vi "Controlador_PID.vi"() -> ()   [LabVIEW 2016]
uses:
  <vilib>/imath/engines/lvmath2/RunTimeEngine/Managers/WorkSpace/UID Generator.vi
  <vilib>/imath/engines/lvmath2/RunTimeEngine/RunTimeType/NIMS_RunTimeType_From StrictType (excl LVString).vi
  <instcachedir>/0/NIMS_RunTimeType_From StrictType (excl LVString)_BBF44FB49F834B71AF7A14CCEDF8BECD.lvgen/NIMS_RunTimeType_From StrictType (excl LVString)_BBF44FB49F834B71AF7A14CCEDF8BECD_000.vi
  <vilib>/imath/engines/lvmath2/RunTimeEngine/LocalVariableDefStatement/MC_LocalVariableDefStatement_Display.vi
  <vilib>/imath/engines/lvmath2/RunTimeEngine/Managers/SymbolTable/Clear UID.vi
  <vilib>/imath/engines/lvmath2/RunTimeEngine/NodeEndStatement/NIMS_NodeEndStatement_Output.vi
  <instcachedir>/0/NIMS_NodeEndStatement_Output_53EC0D466D134D7ABD903AC30B43404B.lvgen/NIMS_NodeEndStatement_Output_53EC0D466D134D7ABD903AC30B43404B_001.vi
  <vilib>/imath/engines/lvmath2/RunTimeEngine/ErrorHandling/NIMS_Finalize Error.vi
  <vilib>/imath/engines/lvmath2/RunTimeEngine/Managers/SymbolTable/NIMS_WorkSpace.lvlib
panel:
  in  "Ki":dbl=1.0
  in  "Kd":dbl=1.0
  in  "Kp":dbl=1.0
  in  "SP":dbl(knob)=1.0 scale=0.0..10.0
  in  "stop":bool
  out "Waveform Chart":cluster{"SP":dbl, "x":dbl}(graph)
  in  "F":dbl=1.0
  in  "k":dbl=1.0
  in  "b":dbl=1.0
  in  "m":dbl=1.0
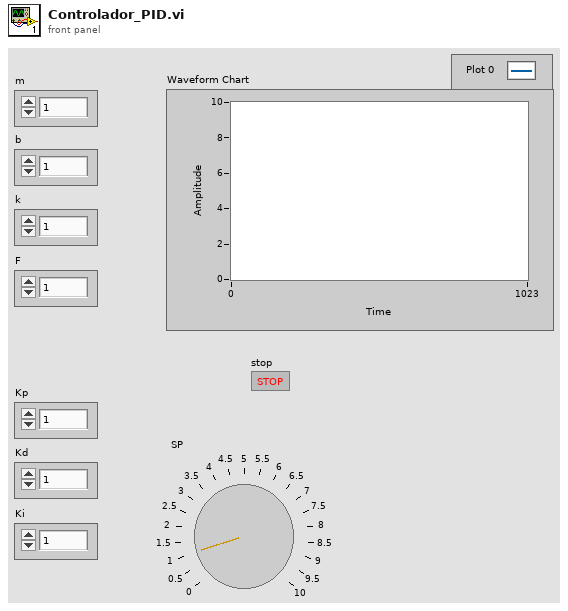
[diagram p1: front panel]
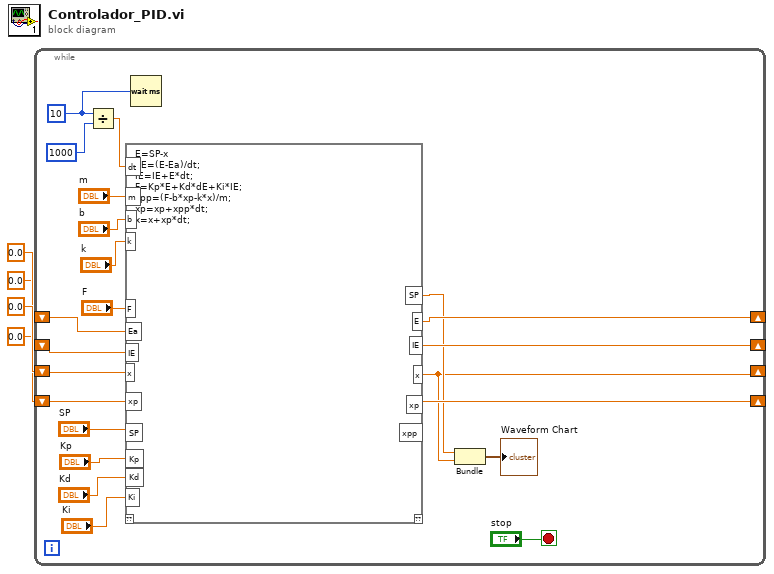
[diagram p0: block diagram]
diagram:
  n1 = while {
    shift-right: [w5] -> _
    shift-left: 0.0 -> [w21]
    shift-right: [w19] -> _
    shift-left: 0.0 -> [w20]
    shift-right: [w9] -> _
    shift-left: 0.0 -> [w10]
    shift-right: [w8] -> _
    shift-left: 0.0 -> [w11]
    stop <- "stop" stop-if-true
    w17 = i16 10 ("x")
    n2 = Divide(x=w17, y=i16 1000) -> (x/y=w16:dbl)
    n3 = mathscript code="E=SP-x\ndE=(E-Ea)/dt;\nIE=IE+E*dt;\nF=Kp*E+Kd*dE+Ki*IE;\nxpp=(F-b*xp-k*x)/m;\nxp=xp+xpp*dt;\nx=x+xp*dt;"("m"="m", "b"="b", "k"="k", "F"="F", "x"=w21, "xp"=w20, "dt"=w16, "SP"="SP", "Kp"="Kp", "Kd"="Kd", "Ki"="Ki", "Ea"=w10, "IE"=w11) -> ("x"=w5:dbl, "xp"=w19:dbl, "E"=w9:dbl, "IE"=w8:dbl, "SP"=w6:dbl)  [unwired: 1 in, 2 out]
    n4 = Wait (ms)(milliseconds to wait=w17) -> ()  [unwired: 1 out]
    n5 = Bundle("SP"=w6, "x"=w5) -> (→"Waveform Chart":cluster{"SP":dbl, "x":dbl})  [unwired: 1 in]
  }
